vi "liczydlo kalkulator.vi"() -> ()   [LabVIEW 2020]
panel:
  in  "Enum":T1(ring)
  out "Wynik (string indicator)":string
  in  "b(numeric control)":dbl
  in  "a(numeric control)":dbl
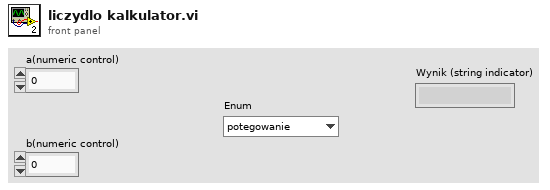
[diagram p1: front panel]
types:
  T1 = enum16{"potegowanie ", "dodawanie", "odejmowanie", "mnozenie", "dzielenie"}
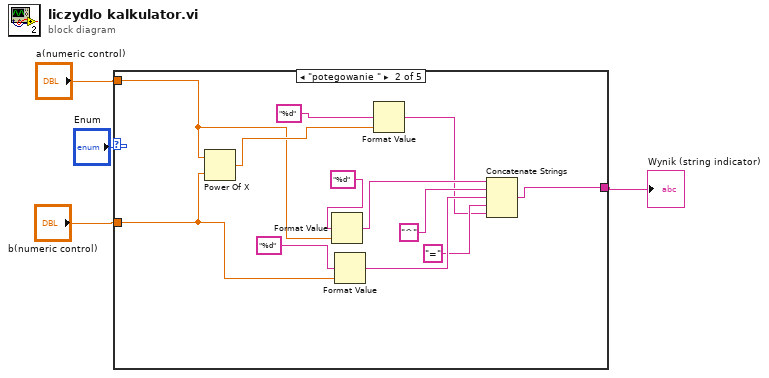
[diagram p0: block diagram]
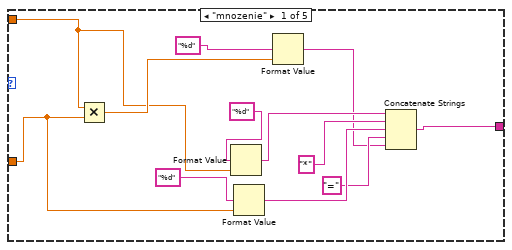
[diagram p2: hidden frame]
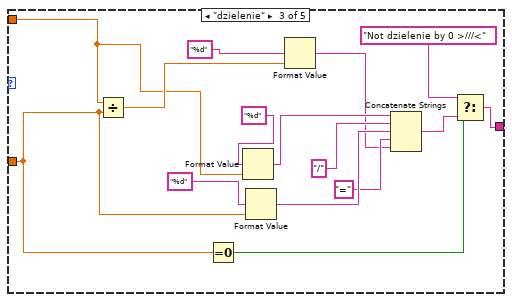
[diagram p3: hidden frame]
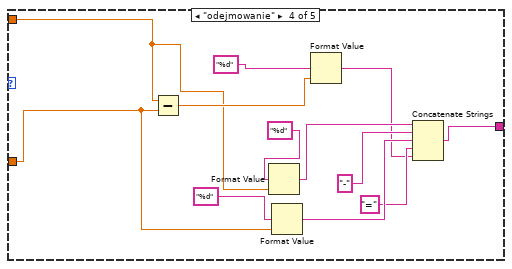
[diagram p4: hidden frame]
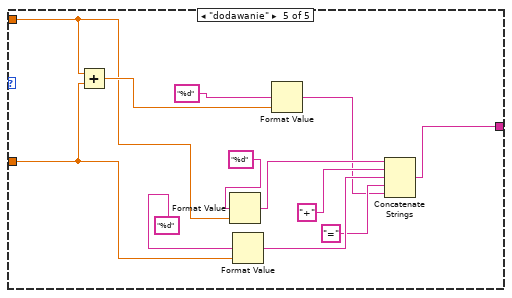
[diagram p5: hidden frame]
diagram:
  n1 = case shown="\"potegowanie \"" "Enum" {
    tunnel: "a(numeric control)" -> [w7 w18 w35 w46 w62]
    tunnel: "b(numeric control)" -> [w5 w17 w33 w44 w66]
    tunnel: [w9 w21 w31 w48 w56] -> w1
    frame "mnozenie" {
      n2 = Multiply(x=w7, y=w5) -> (x*y=w8:dbl)
      n3 = Format Value(format string="%d", value (0)=w7) -> (output string=w14:string)  [unwired: 1 in]
      n4 = Format Value(format string="%d", value (0)=w5) -> (output string=w13:string)  [unwired: 1 in]
      n5 = Format Value(format string="%d", value (0)=w8) -> (output string=w10:string)  [unwired: 1 in]
      n6 = Concatenate Strings(w14, "*", w13, "=", w10) -> (w9:string)
    }
    frame "potegowanie " {
      n7 = Power Of X(1:w17, 2:w18) -> (0:w20:dbl)
      n8 = Format Value(format string="%d", value (0)=w18) -> (output string=w26:string)  [unwired: 1 in]
      n9 = Format Value(format string="%d", value (0)=w17) -> (output string=w25:string)  [unwired: 1 in]
      n10 = Format Value(format string="%d", value (0)=w20) -> (output string=w22:string)  [unwired: 1 in]
      n11 = Concatenate Strings(w26, "^", w25, "=", w22) -> (w21:string)
    }
    frame "dzielenie" {
      n12 = Divide(x=w35, y=w33) -> (x/y=w36:dbl)
      n13 = Equal To 0?(x=w33) -> (x = 0?=w32:bool)
      n14 = Format Value(format string="%d", value (0)=w35) -> (output string=w41:string)  [unwired: 1 in]
      n15 = Format Value(format string="%d", value (0)=w33) -> (output string=w40:string)  [unwired: 1 in]
      n16 = Format Value(format string="%d", value (0)=w36) -> (output string=w37:string)  [unwired: 1 in]
      n17 = Concatenate Strings(w41, "/", w40, "=", w37) -> (w30:string)
      n18 = Select(t="Not dzielenie by 0 >///<", s=w32, f=w30) -> (s? t:f=w31:string)
    }
    frame "odejmowanie" {
      n19 = Subtract(x=w46, y=w44) -> (x-y=w47:dbl)
      n20 = Format Value(format string="%d", value (0)=w46) -> (output string=w53:string)  [unwired: 1 in]
      n21 = Format Value(format string="%d", value (0)=w44) -> (output string=w52:string)  [unwired: 1 in]
      n22 = Format Value(format string="%d", value (0)=w47) -> (output string=w49:string)  [unwired: 1 in]
      n23 = Concatenate Strings(w53, "-", w52, "=", w49) -> (w48:string)
    }
    frame "dodawanie" {
      n24 = Add(x=w62, y=w66) -> (x+y=w67:dbl)
      n25 = Format Value(format string="%d", value (0)=w62) -> (output string=w61:string)  [unwired: 1 in]
      n26 = Format Value(format string="%d", value (0)=w66) -> (output string=w60:string)  [unwired: 1 in]
      n27 = Format Value(format string="%d", value (0)=w67) -> (output string=w57:string)  [unwired: 1 in]
      n28 = Concatenate Strings(w61, "+", w60, "=", w57) -> (w56:string)
    }
  }
  "Wynik (string indicator)" <- w1
